vi "MatrixConfiguration.vi"() -> ()   [LabVIEW 2018]
uses:
  InstrControl/Switching/Switching.lvclass
  InstrControl/Switching/Pickering/Pickering.lvclass
  InstrControl/InstrumentSetup.vi
  globals/QC_RunInformation.vi
  InstrControl/InstrControl.lvclass
panel:
  in  "DUT Switch":string(combo)="Keithley 3706A"
  in  "Measurement Switch":string(combo)="Pickering Matrix"
  in  "OK Button":bool
  in  "No Measurement\nSwitch":bool=TRUE
  in  "Tab Control":enum32{"Pickering Matrix", "Keithley 3706A"}(tab)
  out "Y Mapping":string[](array[string])
  out "X Mapping":string[](array[string])
  out "Display Pickering Matrix":bool[][](array[boolean])
  out "DIAGNOSTIC? Response":string
  in  "Pickering DIAGNOSTIC?":bool
  in  "Pickering Mux2 address":string caption="Mux2 address"
  in  "Pickering Mux1 address":string caption="Mux1 address"
  in  "Pickering address":refnum<visa-resource-name> caption="Crate address"
  in  "Pickering Matrix address":string caption="Matrix address"
  out "X Mapping CB Standard":string[](array[string])
  in  "Apply":bool
  in  "Pickering Measurement":T1(ring)
  out "KE3706A slot occupation":string[](array[string])
  out "KE3706A card occupation":string[](array[string])
  in  "KE3706A Mux2 address":string caption="Mux2 slot"
  in  "KE3706A Mux1 address":string caption="Mux1 slot"
  in  "Keithley 3706A address":refnum<visa-resource-name>
  # "MUX / Matrix Setup"
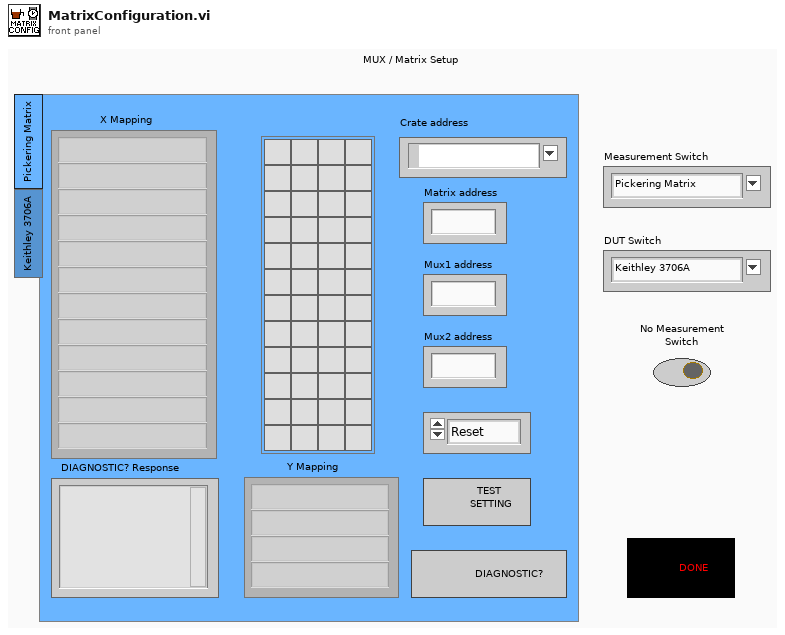
[diagram p1: front panel]
types:
  T1 = enum16{"Reset", "IV", "CV", "Stability", "Striptest", "Cis", "Ris", "PTP"}
  T2 = enum16{"Reset", "Ground", "Striptest SMU", "Striptest LCR", "IV", "CV", "Interstrip Cap", "Interstrip Res"}
  T3 = cluster{"Matrix address":string, "Mux1 address":string, "Mux2 address":string, "Pickering":refnum<class "Pickering.lvclass">, "Matrix X Channels":cluster{"Bias Supply / SMU LO":i32, "Bias Supply / SMU HI":i32, "CV Box LO":i32, "CV Box HI":i32, "CV Box LO IN":i32, "CV Box HI IN":i32, "Volt meter LO":i32, "Volt meter HI":i32, "Mux1 C1":i32, "Mux1 C2":i32, "Mux2 C1":i32, "Mux2 C2":i32}}
  T4 = cluster{"KE 2410":cluster{"Instrument name":string, "address":refnum<visa-resource-name>, "Instrument type":u16}, "KE 6517":cluster{"Instrument name":string, "address":refnum<visa-resource-name>, "Instrument type":u16}, "KE 487":cluster{"Instrument name":string, "address":refnum<visa-resource-name>, "Instrument type":u16}, "KE 236":cluster{"Instrument name":string, "address":refnum<visa-resource-name>, "Instrument type":u16}, "WK 6440B":cluster{"Instrument name":string, "address":refnum<visa-resource-name>, "Instrument type":u16}, "WK 6425":cluster{"Instrument name":string, "address":refnum<visa-resource-name>, "Instrument type":u16}, "Pickering Matrix":cluster{"Instrument name":string, "address":refnum<visa-resource-name>, "Instrument type":u16}, "KE 2000":cluster{"Instrument name":string, "address":refnum<visa-resource-name>, "Instrument type":u16}, "KE3706A Switching":cluster{"Instrument name":string, "address":refnum<visa-resource-name>, "Instrument type":u16}, "HP 4284A":cluster{"Instrument name":string, "address":refnum<visa-resource-name>, "Instrument type":u16}, "KE237":cluster{"Instrument name":string, "address":refnum<visa-resource-name>, "Instrument type":u16}}
  T5 = cluster{"Mux1 slot":string, "Mux2 slot":string, "KE3706A":refnum<class "KE3706A.lvclass">}
  T6 = enum16{"Left Button", "Center Button", "Right Button", "Window Close"}
  T7 = cluster{"Institute":string, "Manufacturers":string[], "Devices":string[], "Serialnumbers Lookup DB":string, "Data directory":string, "Backup & screenshot directory":string, "List of known users":string[], "Measurement switch not used":bool, "Measurement Switch":string, "DUT Switch":string, "Rseries IV [MOhm]":string, "Rshunt IV [MOhm]":string, "Rseries CV [MOhm]":string, "DC blocking Cap [µF]":string, "Rseries LCR [MOhm]":string, "Rseries stability [MOhm]":string, "Rshunt stability [MOhm]":string, "Rseries striptest bias [MOhm]":string, "Rseries strip pinhole [MOhm]":string}
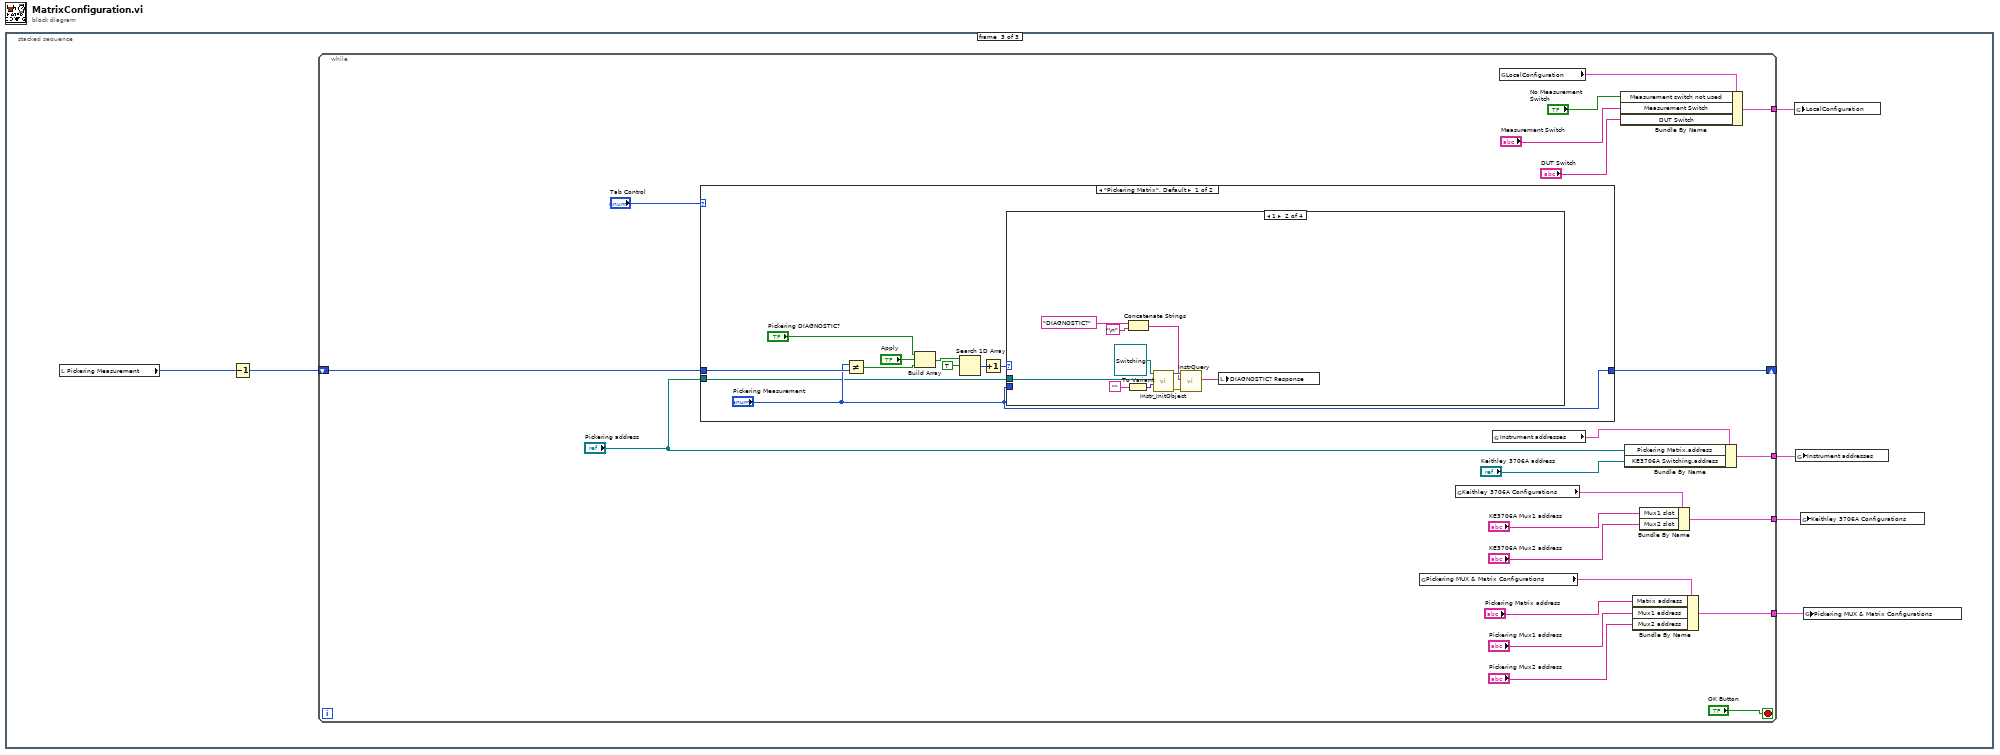
[diagram p0: block diagram]
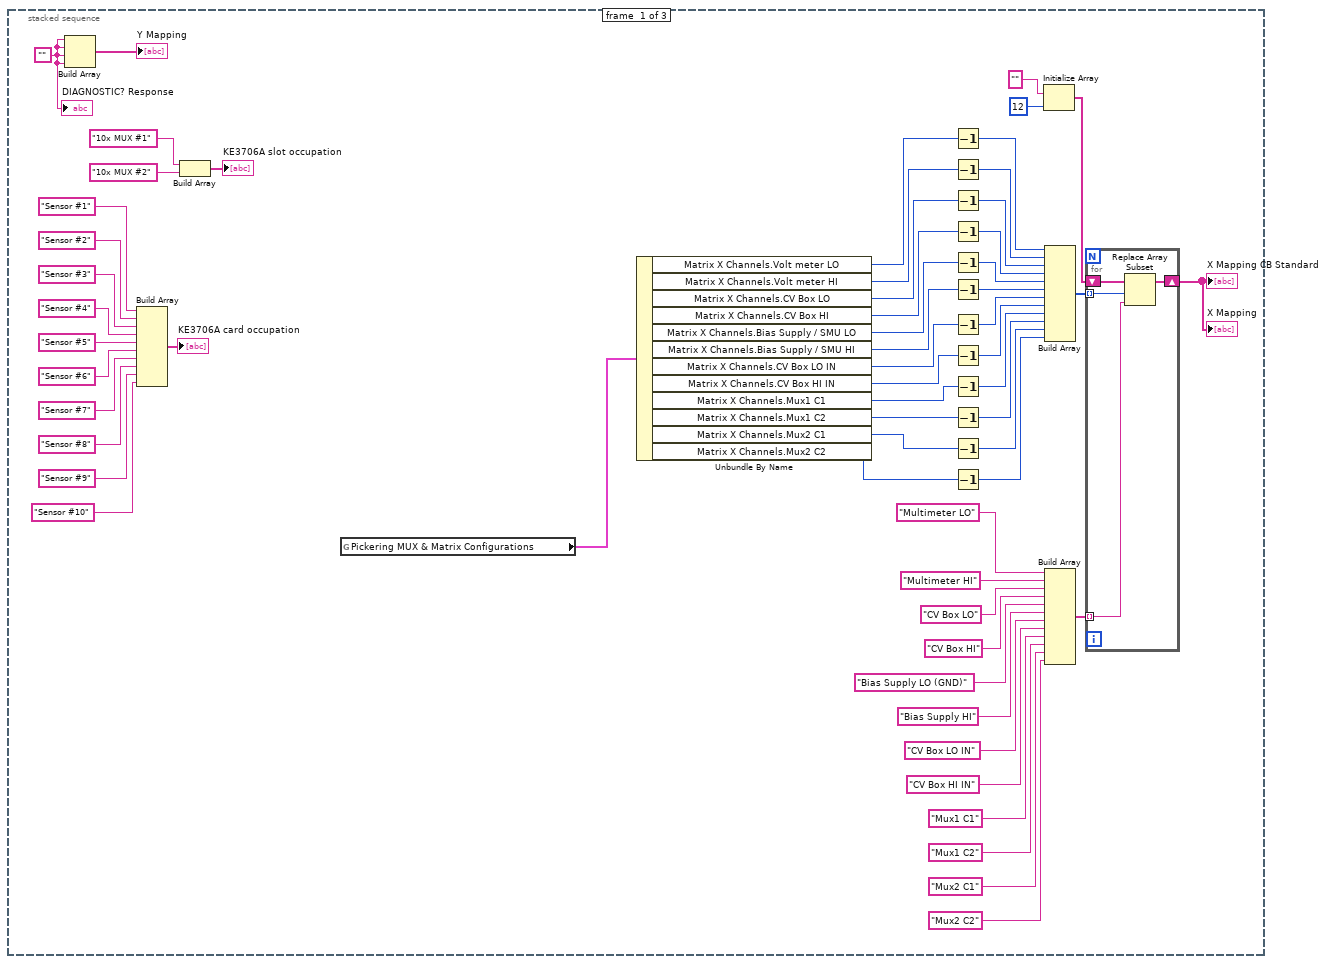
[diagram p2: hidden frame]
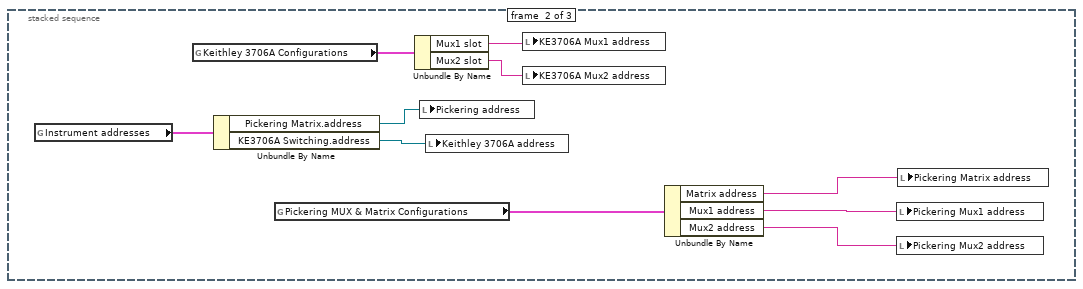
[diagram p3: hidden frame]
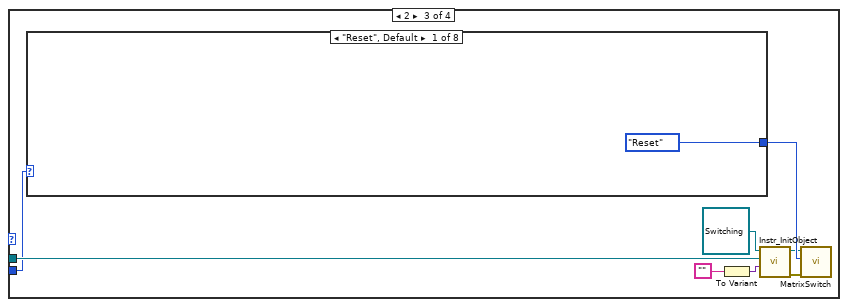
[diagram p5: hidden frame]
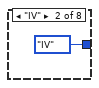
[diagram p6: hidden frame]
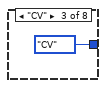
[diagram p7: hidden frame]
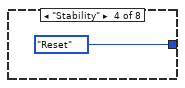
[diagram p8: hidden frame]
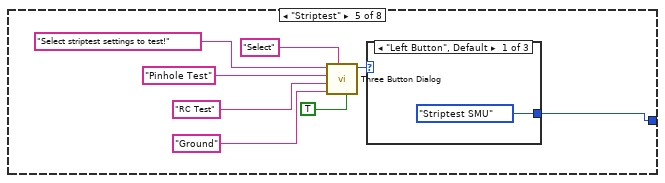
[diagram p9: hidden frame]
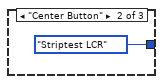
[diagram p10: hidden frame]
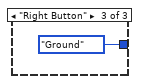
[diagram p11: hidden frame]
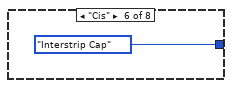
[diagram p12: hidden frame]
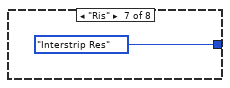
[diagram p13: hidden frame]
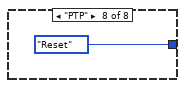
[diagram p14: hidden frame]
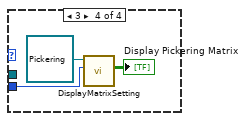
[diagram p15: hidden frame]
diagram:
  n1 = stacked-sequence {
    frame #0 {
      w15 = ""
      n2 = Build Array(w15, w15, w15, w15) -> (→"Y Mapping":string[])
      n3 = Build Array("Sensor #1" ("Input Element"), "Sensor #2" ("Input Element"), "Sensor #3" ("Input Element"), "Sensor #4" ("Input Element"), "Sensor #5" ("Input Element"), "Sensor #6" ("Input Element"), "Sensor #7" ("Input Element"), "Sensor #8" ("Input Element"), "Sensor #9" ("Input Element"), "Sensor #10" ("Input Element")) -> (→"KE3706A card occupation":string[])
      n4 = Build Array("10x MUX #1" ("Input Element"), "10x MUX #2" ("Input Element")) -> (→"KE3706A slot occupation":string[])
      n5 = global read "InstrumentSetup.vi" "Pickering MUX & Matrix Configurations"() -> (w31:T3)
      n6 = Unbundle By Name(w31) -> ("Matrix X Channels.Volt meter LO"=w41:i32, "Matrix X Channels.Volt meter HI"=w43:i32, "Matrix X Channels.CV Box LO"=w32:i32, "Matrix X Channels.CV Box HI"=w37:i32, "Matrix X Channels.Bias Supply / SMU LO"=w36:i32, "Matrix X Channels.Bias Supply / SMU HI"=w35:i32, "Matrix X Channels.CV Box LO IN"=w34:i32, "Matrix X Channels.CV Box HI IN"=w33:i32, "Matrix X Channels.Mux1 C1"=w40:i32, "Matrix X Channels.Mux1 C2"=w39:i32, "Matrix X Channels.Mux2 C1"=w38:i32, "Matrix X Channels.Mux2 C2"=w18:i32)
      n7 = Decrement(x=w41) -> (x-1=w42:i32)
      n8 = Decrement(x=w43) -> (x-1=w44:i32)
      n9 = Decrement(x=w32) -> (x-1=w45:i32)
      n10 = Decrement(x=w37) -> (x-1=w46:i32)
      n11 = Decrement(x=w36) -> (x-1=w47:i32)
      n12 = Decrement(x=w35) -> (x-1=w48:i32)
      n13 = Decrement(x=w34) -> (x-1=w49:i32)
      n14 = Decrement(x=w33) -> (x-1=w50:i32)
      n15 = Decrement(x=w40) -> (x-1=w51:i32)
      n16 = Decrement(x=w39) -> (x-1=w52:i32)
      n17 = Decrement(x=w38) -> (x-1=w53:i32)
      n18 = Decrement(x=w18) -> (x-1=w54:i32)
      n19 = Initialize Array("", 12) -> (w59:string[])
      n20 = Build Array(w42, w44, w45, w46, w47, w48, w49, w50, w51, w52, w53, w54) -> (w55:i32[])
      n21 = Build Array("Multimeter LO" ("Input Element"), "Multimeter HI" ("Input Element"), "CV Box LO" ("Input Element"), "CV Box HI" ("Input Element"), "Bias Supply LO (GND)" ("Input Element"), "Bias Supply HI" ("Input Element"), "CV Box LO IN" ("Input Element"), "CV Box HI IN" ("Input Element"), "Mux1 C1" ("String"), "Mux1 C2" ("String"), "Mux2 C1" ("String"), "Mux2 C2" ("String")) -> (w56:string[])
      n22 = for {
        tunnel: w55 -> [w61] mode=indexing
        tunnel: w56 -> [w62] mode=indexing
        shift-right: [w60] -> w17
        shift-left: w59 -> [w63]
        n23 = Replace Array Subset(array=w63, new element=w62, index=w61) -> (w60:string[])
      }
      "X Mapping" <- w17
      "X Mapping CB Standard" <- w17
      "DIAGNOSTIC? Response" <- w15
    }
    frame #1 {
      n24 = global read "InstrumentSetup.vi" "Instrument addresses"() -> (w66:T4)
      n25 = global read "InstrumentSetup.vi" "Keithley 3706A Configurations"() -> (w69:T5)
      n26 = Unbundle By Name(w66) -> ("Pickering Matrix.address"=w65:refnum<visa-resource-name>, "KE3706A Switching.address"=w64:refnum<visa-resource-name>)
      n27 = global read "InstrumentSetup.vi" "Pickering MUX & Matrix Configurations"() -> (w73:T3)
      n28 = Unbundle By Name(w69) -> ("Mux1 slot"=w68:string, "Mux2 slot"=w67:string)
      n29 = local write "Pickering address"(w65) -> ()
      n30 = local write "Keithley 3706A address"(w64) -> ()
      n31 = local write "KE3706A Mux1 address"(w68) -> ()
      n32 = local write "KE3706A Mux2 address"(w67) -> ()
      n33 = Unbundle By Name(w73) -> ("Matrix address"=w72:string, "Mux1 address"=w71:string, "Mux2 address"=w70:string)
      n34 = local write "Pickering Mux1 address"(w71) -> ()
      n35 = local write "Pickering Mux2 address"(w70) -> ()
      n36 = local write "Pickering Matrix address"(w72) -> ()
    }
    frame #2 {
      n37 = local read "Pickering Measurement"() -> (w79:T1)
      n38 = Decrement(x=w79) -> (x-1=w78:T1)
      n39 = while {
        shift-right: [w100] -> _
        shift-left: w78 -> [w101]
        tunnel: [w89] -> w77
        tunnel: [w87] -> w76
        tunnel: [w81] -> w75
        tunnel: [w80] -> w74
        stop <- "OK Button" stop-if-true
        n40 = case shown="\"Pickering Matrix\", Default" "Tab Control" {
          tunnel: w101 -> [w110 w151]
          tunnel: ["Pickering Measurement" w151] -> w100
          tunnel: "Pickering address" -> [w102 _]
          frame "Pickering Matrix", Default {
            n41 = Not Equal?(x="Pickering Measurement", y=w110) -> (x != y?=w111:bool)
            n42 = Build Array("Pickering DIAGNOSTIC?", "Apply", w111) -> (w106:bool[])
            n43 = Search 1D Array(1D array=w106, element=TRUE) -> (index of element=w108:i32)  [unwired: 1 in]
            n44 = Increment(x=w108) -> (x+1=w105:i32)
            n45 = case shown="1" w105 {
              tunnel: w102 -> [_ w115 w128 _]
              tunnel: "Pickering Measurement" -> [_ _ w122 w150]
              frame 0, Default {
              }
              frame 1 {
                n46 = To Variant(anything="") -> (Variant=w120:variant)
                n47 = Concatenate Strings("DIAGNOSTIC?", "\n") -> (w112:string)
                n48 = call-dynamic "Instr_InitObject.vi"("Instrument Configuration"=w120, "Instrument address"=w115, "Switching in"=refnum<class "Switching.lvclass"> refnum ("Switching.lvclass")) -> ("error out"=w118:errorcluster, "Switching out"=w117:refnum<class "Switching.lvclass">)  [unwired: 7 in]
                n49 = call-dynamic "InstrQuery.vi"("error in (no error)"=w118, "Command string"=w112, "InstControl in"=w117) -> ("Instrument response"=w121:string)  [unwired: 6 in, 2 out]
                n50 = local write "DIAGNOSTIC? Response"(w121) -> ()
              }
              frame 2 {
                n51 = case shown="\"Reset\", Default" w122 {
                  tunnel: [T2."Reset" ("Action") T2."IV" ("Action") T2."CV" ("Action") T2."Reset" ("Action") w139 T2."Interstrip Cap" ("Action") T2."Interstrip Res" ("Action") T2."Reset" ("Action")] -> w127
                  frame "Reset", Default {
                  }
                  frame "IV" {
                  }
                  frame "CV" {
                  }
                  frame "Stability" {
                  }
                  frame "Striptest" {
                    n52 = call <vilib>:"Three Button Dialog.vi"("Allow user to close window? (TRUE)"=TRUE, "Window Title (\"\")"="Select", "Right Button Text (\"Cancel\")"="Ground", "Center Button Text (\"No\")"="RC Test", "Left Button Text (\"Yes\")"="Pinhole Test", "message"="Select striptest settings to test!") -> ("Which Button?"=w141:T6)  [unwired: 5 in]
                    n53 = case shown="\"Left Button\", Default" w141 {
                      tunnel: [T2."Striptest SMU" ("Action") T2."Striptest LCR" ("Action") T2."Ground" ("Action")] -> w139
                      frame "Left Button", Default {
                      }
                      frame "Center Button" {
                      }
                      frame "Right Button" {
                      }
                    }
                  }
                  frame "Cis" {
                  }
                  frame "Ris" {
                  }
                  frame "PTP" {
                  }
                }
                n54 = To Variant(anything="") -> (Variant=w123:variant)
                n55 = call-dynamic "Instr_InitObject.vi"("Instrument Configuration"=w123, "Instrument address"=w128, "Switching in"=refnum<class "Switching.lvclass"> refnum) -> ("error out"=w125:errorcluster, "Switching out"=w126:refnum<class "Switching.lvclass">)  [unwired: 7 in]
                n56 = call-dynamic "MatrixSwitch.vi"("error in (no error)"=w125, "Action"=w127, "Switching in"=w126) -> ()  [unwired: 6 in, 3 out]
              }
              frame 3 {
                n57 = call "DisplayMatrixSetting.vi"("Measurement"=w150, "Pickering in"=refnum<class "Pickering.lvclass"> refnum) -> ("Display Pickering Matrix"=→"Display Pickering Matrix":bool[][])  [unwired: 7 in, 2 out]
              }
            }
          }
          frame "Keithley 3706A" {
          }
        }
        n58 = global read "InstrumentSetup.vi" "Pickering MUX & Matrix Configurations"() -> (w97:T3)
        n59 = global read "InstrumentSetup.vi" "Keithley 3706A Configurations"() -> (w84:T5)
        n60 = global read "InstrumentSetup.vi" "Instrument addresses"() -> (w88:T4)
        n61 = global read "QC_RunInformation.vi" "LocalConfiguration"() -> (w93:T7)
        n62 = Bundle By Name(cluster=w93, "Measurement switch not used"="No Measurement\nSwitch", "Measurement Switch"="Measurement Switch", "DUT Switch"="DUT Switch") -> (w89:T7)
        n63 = Bundle By Name(cluster=w88, "Pickering Matrix.address"="Pickering address", "KE3706A Switching.address"="Keithley 3706A address") -> (w87:T4)
        n64 = Bundle By Name(cluster=w97, "Matrix address"="Pickering Matrix address", "Mux1 address"="Pickering Mux1 address", "Mux2 address"="Pickering Mux2 address") -> (w81:T3)
        n65 = Bundle By Name(cluster=w84, "Mux1 slot"="KE3706A Mux1 address", "Mux2 slot"="KE3706A Mux2 address") -> (w80:T5)
      }
      n66 = global write "QC_RunInformation.vi" "LocalConfiguration"(w77) -> ()
      n67 = global write "InstrumentSetup.vi" "Instrument addresses"(w76) -> ()
      n68 = global write "InstrumentSetup.vi" "Keithley 3706A Configurations"(w74) -> ()
      n69 = global write "InstrumentSetup.vi" "Pickering MUX & Matrix Configurations"(w75) -> ()
    }
  }
